vi "Setintf_ref_array.vi"(8 "error in (no error)":errorcluster, 10 "Set_Val":T1, 11 "OneOfTemplate in":refnum<class "nixnet_grpc_GetPropertyResponse_property_value.lvclass">) -> (0 "error out":errorcluster, 3 "OneOfTemplate out":refnum<class "nixnet_grpc_GetPropertyResponse_property_value.lvclass">)   [LabVIEW 2019, in "grpc-xnet_client.lvlib" / "nixnet_grpc_GetPropertyResponse_property_value.lvclass"]
uses:
  nixnet_grpc_GetPropertyResponse_property_value.lvclass
  nixnet_grpc_InterfaceRefArray.ctl
  nidevice_grpc_Session.ctl
  nixnet_grpc_GetPropertyResponse_property_value.lvclass/nixnet_grpc_GetPropertyResponse_property_value.ctl
  grpc-xnet_client.lvlib
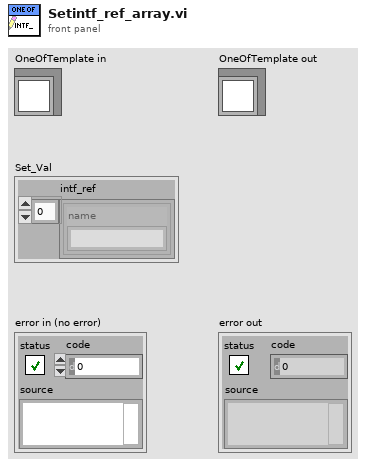
[diagram p1: front panel]
types:
  T1 = typedef "grpc-xnet_client.lvlib/nixnet_grpc_InterfaceRefArray.ctl" = cluster{"intf_ref":T2[]}
  T2 = typedef "grpc-xnet_client.lvlib/nidevice_grpc_Session.ctl" = cluster{"name":string}
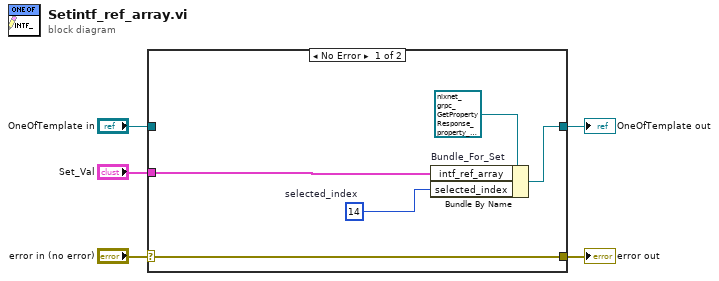
[diagram p0: block diagram]
diagram:
  n1 = case shown="No Error" "error in (no error)" {
    selector: "error in (no error)" -> [w10 w11]
    tunnel: [w10 w11] -> w4
    tunnel: [w9 w12] -> w2
    tunnel: "OneOfTemplate in" -> [_ w12]
    tunnel: "Set_Val" -> [w8 _]
    frame No Error {
      w7 = 14  # selected_index
      n2 = Bundle By Name "Bundle_For_Set"(cluster=refnum<class "nixnet_grpc_GetPropertyResponse_property_value.lvclass"> refnum ("OneOfTemplate in"), "intf_ref_array"=w8, "selected_index"=w7) -> (w9:refnum<class "nixnet_grpc_GetPropertyResponse_property_value.lvclass">)
    }
    frame Error {
    }
  }
  "error out" <- w4
  "OneOfTemplate out" <- w2
